vi "Calibrate Offset Data Query.vi"(6 "Filter":i32(ring) caption="Lowpass Filter" items=["Bypass", "Lowpass"], 7 "Impedance":dbl(ring) items=["50 Ohm", "1 MOhm"], 8 "error in":errorcluster, 9 "Range":dbl, 10 "Input Channel":i32(ring) caption="Channel" items=["Input Channel 1", "Input Channel 2", "Input Channel 3", "Input Channel 4"], 11 "Instrument Handle In":i32) -> (0 "error out":errorcluster, 1 "Gain Code":u16, 2 "Zero Code":u16, 3 "Instrument Handle Out":i32)   [LabVIEW 8.6, in "ZTScopeM.lvlib"]
doc: "Query the instrument's offset calibration settings. See the instrument calibration manual for more information."
uses:
  ZTScopeM.lvlib
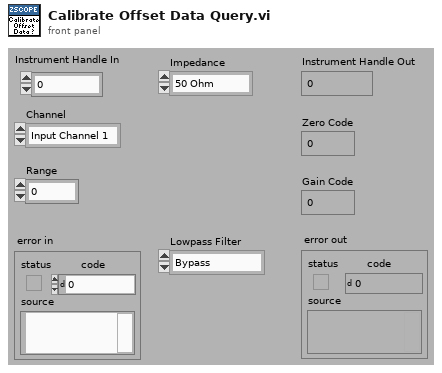
[diagram p1: front panel]
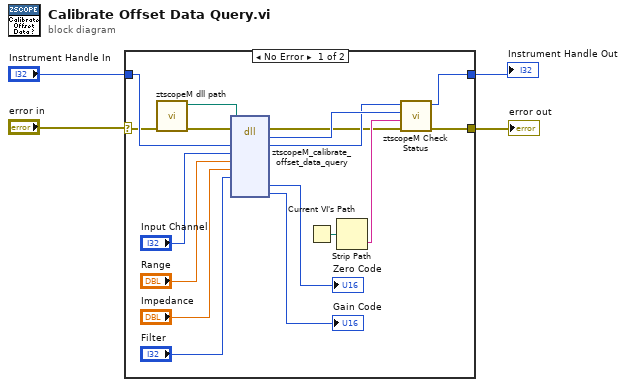
[diagram p0: block diagram]
diagram:
  n1 = case shown="No Error" "error in" {
    selector: "error in" -> [w8 w23]
    tunnel: [w16 w23] -> w1
    tunnel: "Instrument Handle In" -> [w21 w22]
    tunnel: [w15 w22] -> w3
    frame #0 {
      n2 = call "ztscopeM dll path.vi"("error in (no error)"=w8) -> ("error out"=w6:errorcluster, "<instrument>.dll path"=w7:path)  [unwired: 9 in]
      n3 = dll-call lib="C:/Program Files (x86)/National Instruments/LabVIEW 2013/instr.lib/ztscopem/ztscopeM.dll" fn="ztscopeM_calibrate_offset_data_query"(path in=w7, error in=w6, "instrumentHandle"=w21, "Channel"="Input Channel", "Range"="Range", "Impedance"="Impedance", "Lowpass Filter"="Filter") -> (error out=w5:errorcluster, w18:i32, "instrumentHandle"=w17:i32, "Offset"=→"Zero Code":u16, "Adjustment"=→"Gain Code":u16)  [unwired: 7 in, 1 out]
      n4 = Current VI's Path() -> (path=w20:path)
      n5 = Strip Path(path=w20) -> (name=w19:string)  [unwired: 1 out]
      n6 = call "ztscopeM Check Status.vi"("error in"=w5, "name of VI"=w19, "status (return code)"=w18, "instrument handle in"=w17) -> ("error out"=w16:errorcluster, "instrument handle out"=w15:i32)  [unwired: 2 in]
    }
    frame #1 {
    }
  }
  "Instrument Handle Out" <- w3
  "error out" <- w1
